vi "Test.vi"   [LabVIEW 2018]
doc: "This VI is called when test mode begins, and will automatically be terminated when it ends. You can add manual or automatic tests and invoke them from the dashboard."
uses:
  <vilib>/Rock Robotics/WPI/ThirdParty/Sensors/navX/_TypeDefs/FRIC_navX_DeviceNumbersTypeDef.ctl
  <vilib>/Rock Robotics/WPI/Utilities/WPI_GetSetVariantRefNum.vi
  <vilib>/Rock Robotics/Network Tables/NT Write Boolean.vi
  Robot Global Data.vi
  <vilib>/Rock Robotics/WPI/RobotDrive/WPI_RobotDriveMecanumDrive_Cartesian.vi
  <vilib>/Rock Robotics/WPI/ThirdParty/Phoenix-LabVIEW/Motor Controller/Get/CTRE_Phoenix_MotorController_GetQuadratureData.vi
  <vilib>/Rock Robotics/WPI/ThirdParty/Sensors/navX/_Processing Loop/FRIC_navX_Internal_Serial_ProcessingLoop.vi
types:
  T1 = typedef "FRIC_navX_DeviceNumbersTypeDef.ctl" = enum16{"Dev0", "Dev1", "Dev2", "Dev3"}
  T2 = cluster{"Yaw":dbl, "Roll":dbl, "Pitch":dbl, "Heading":dbl, "Fused Heading":dbl}
  T3 = typedef "WPI_JoystickDevRef.ctl" = cluster{"Device":T4}
  T4 = typedef "WPI_JoystickDeviceEnum.ctl" = enum16{"USB 0", "USB 1", "USB 2", "USB 3", "USB 4", "USB 5"}
  T5 = typedef "WPI_RobotDriveDevRef.ctl" = cluster{"DevStatus":errorcluster, "Motors[]":T6[], "Square Inputs":bool, "Max Output":dbl}
  T6 = typedef "WPI_MotorControlDeviceRef.ctl" = cluster{"DeviceStatus":errorcluster, "Type":T7, "PWM":cluster{"PWM Channel":T8, "DeadBand":T9}, "CAN":cluster{"Device Number":u8, "SetOutput VI Ref":variant, "GetOutput VI Ref":variant, "Enable VI Ref":variant, "Disable VI Ref":variant, "Data":variant}, "Invert":bool, "DIO PWM":cluster{"PWM \"Enable\" Channel":T8, "DIOChannel":T10, "PWM Rate":dbl}}
  T7 = typedef "WPI_MotorControlType.ctl" = enum16{"PWM", "CAN", "DIO PWM"}
  T8 = typedef "FPGA_DIOPWMChannel.ctl" = enum8{"PWM 0", "PWM 1", "PWM 2", "PWM 3", "PWM 4", "PWM 5", "PWM 6", "PWM 7", "PWM 8", "PWM 9", "PWM MXP 0", "PWM MXP 1", "PWM MXP 2", "PWM MXP 3", "PWM MXP 4", "PWM MXP 5", "PWM MXP 6", "PWM MXP 7", "PWM MXP 8", "PWM MXP 9", "Invalid"}
  T9 = typedef "WPI_PWMDeadband.ctl" = cluster{"Name":string, "maxPositivePwm":i32, "minPositivePwm":i32, "centerPwm":i32, "maxNegativePwm":i32, "minNegativePwm":i32, "angularRange":u16}
  T10 = typedef "FPGA_DIOChannel.ctl" = enum8{"DIO 0", "DIO 1", "DIO 2", "DIO 3", "DIO 4", "DIO 5", "DIO 6", "DIO 7", "DIO 8", "DIO 9", "DIO MXP 0", "DIO MXP 1", "DIO MXP 2", "DIO MXP 3", "DIO MXP 4", "DIO MXP 5", "DIO MXP 6", "DIO MXP 7", "DIO MXP 8", "DIO MXP 9", "DIO MXP 10", "DIO MXP 11", "DIO MXP 12", "DIO MXP 13", "DIO MXP 14", "DIO MXP 15", "SPI Port CS1", "SPI Port CS2", "SPI Port CS3", "SPI Port MISO", "SPI Port MOSI", "Invalid"}
  T11 = typedef "WPI_SwitchDevRef.ctl" = cluster{"DevStatus":errorcluster, "DIO Channel":T10, "CntIndex":T12, "Normally Closed":bool}
  T12 = typedef "FPGA_CounterCtrSystemIndex.ctl" = enum8{"Ctr 0", "Ctr 1", "Ctr 2", "Ctr 3", "Ctr 4", "Ctr 5", "Ctr 6", "Ctr 7", "Invalid"}
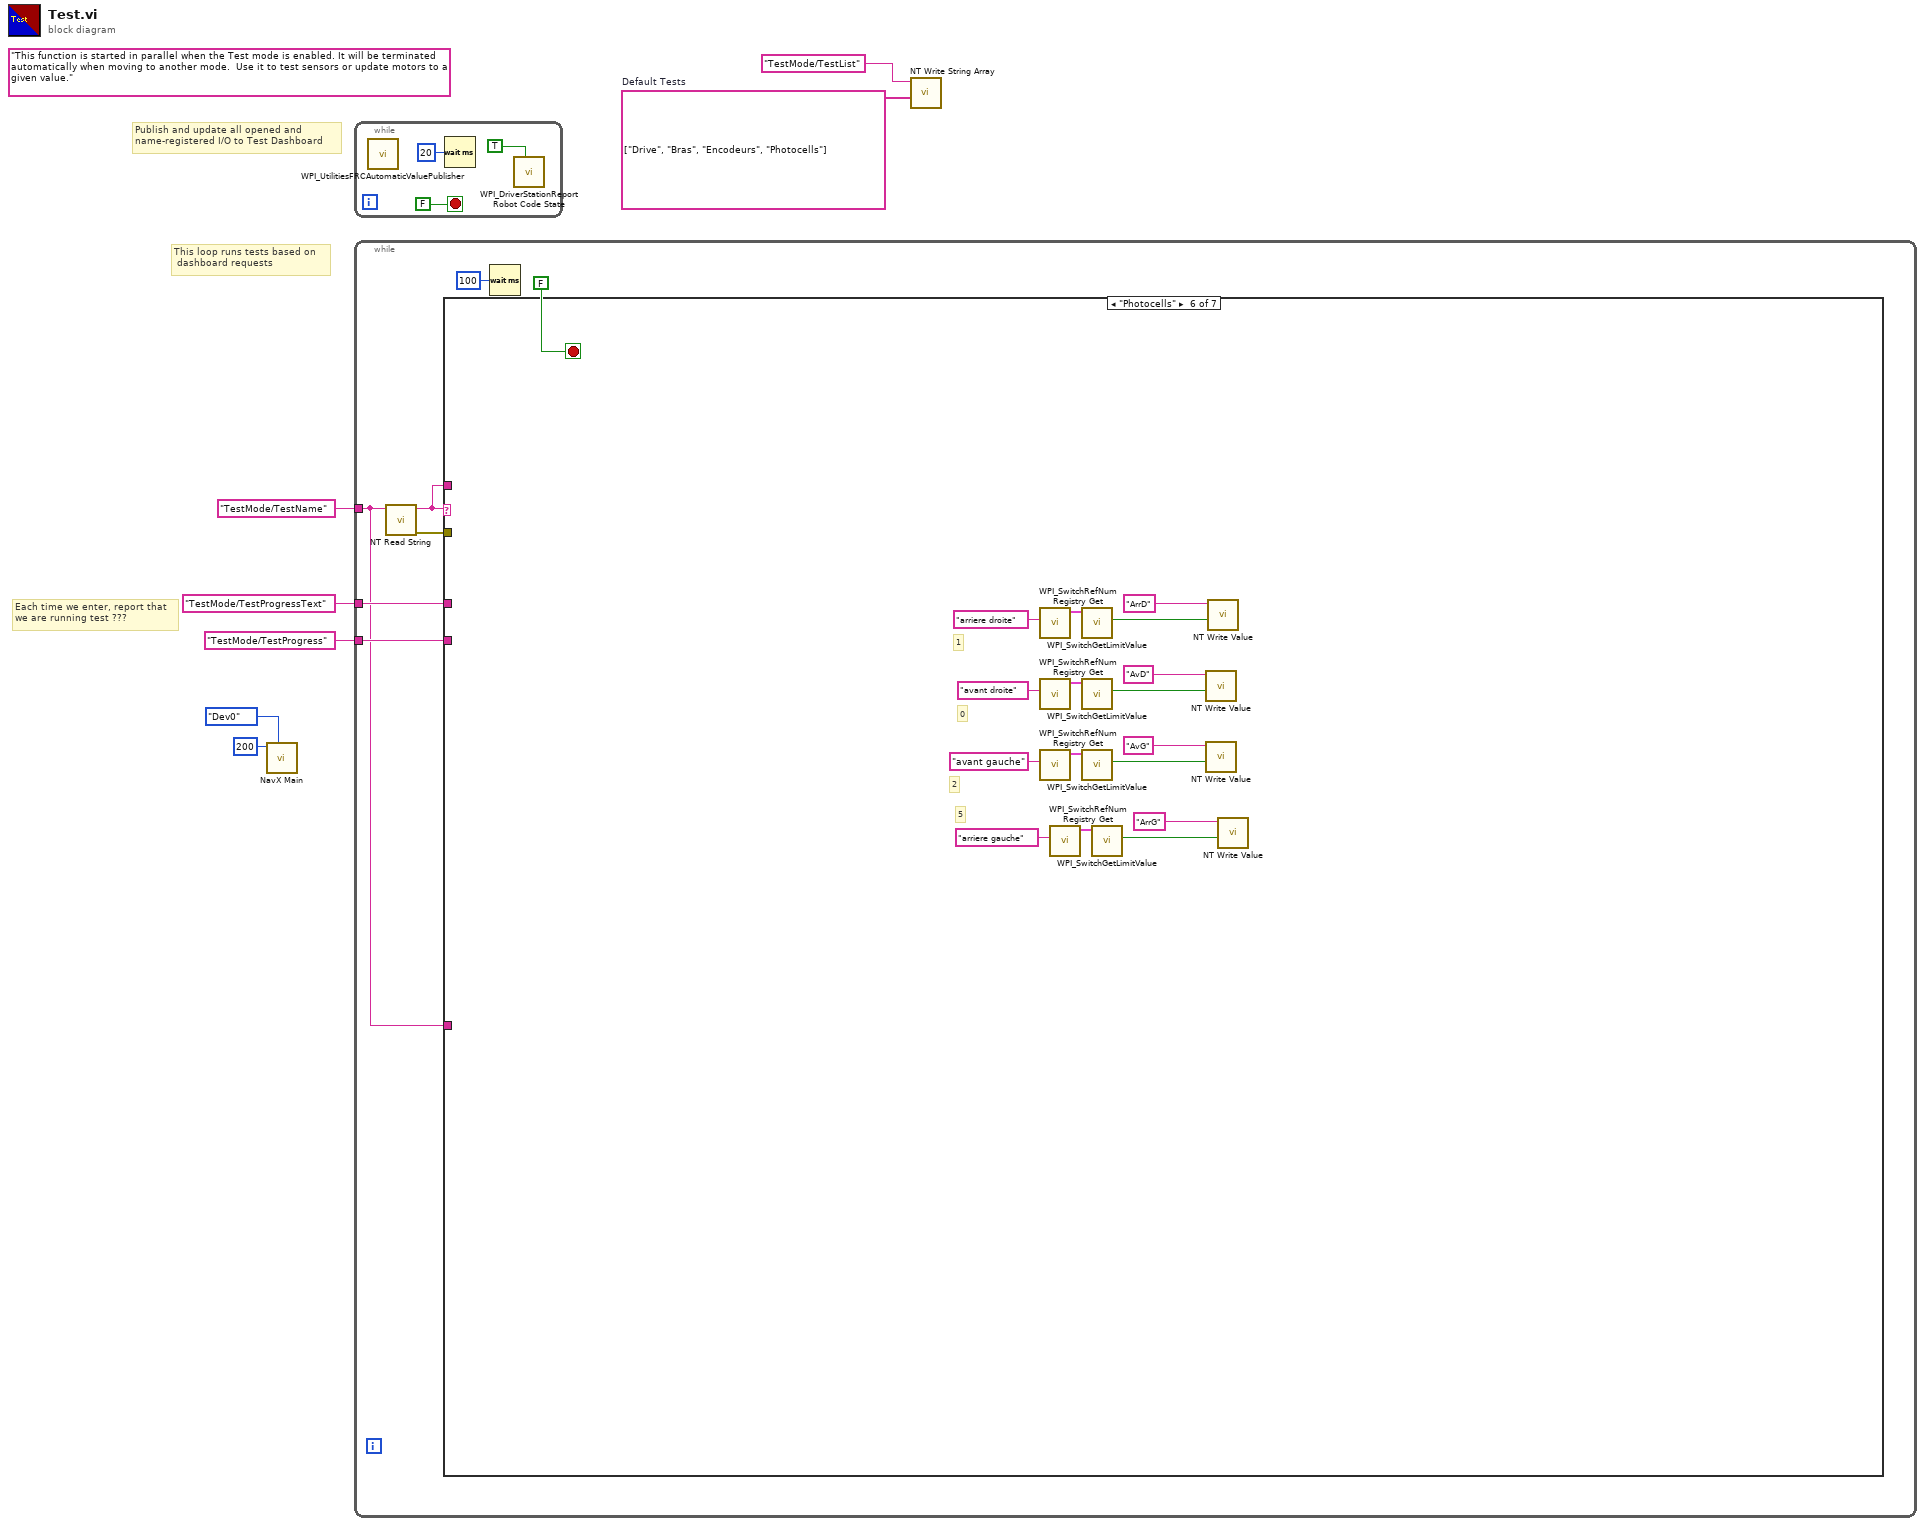
[diagram p0: block diagram]
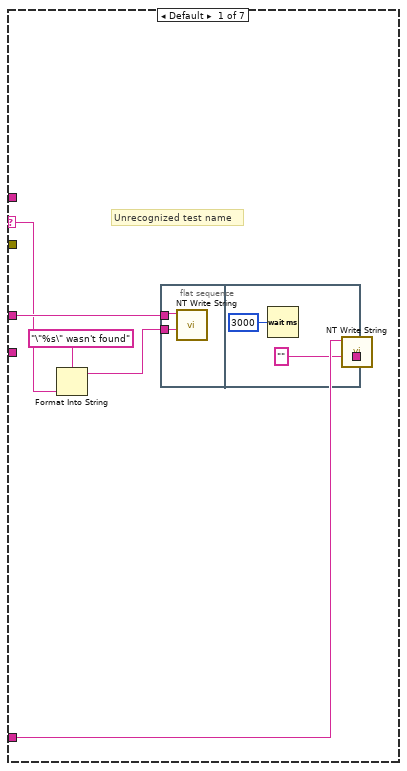
[diagram p2: hidden frame]
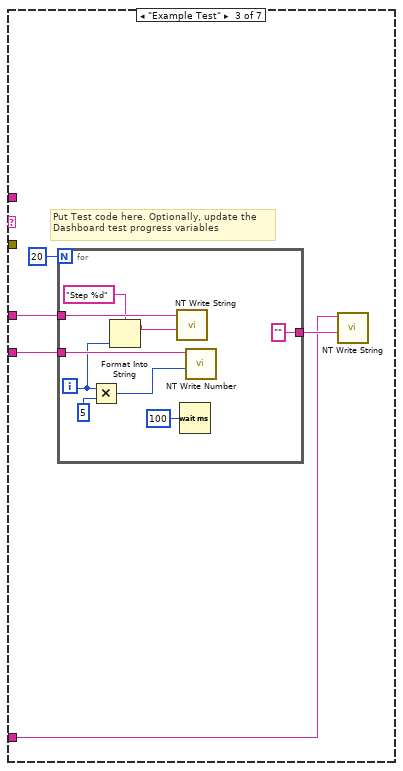
[diagram p4: hidden frame]
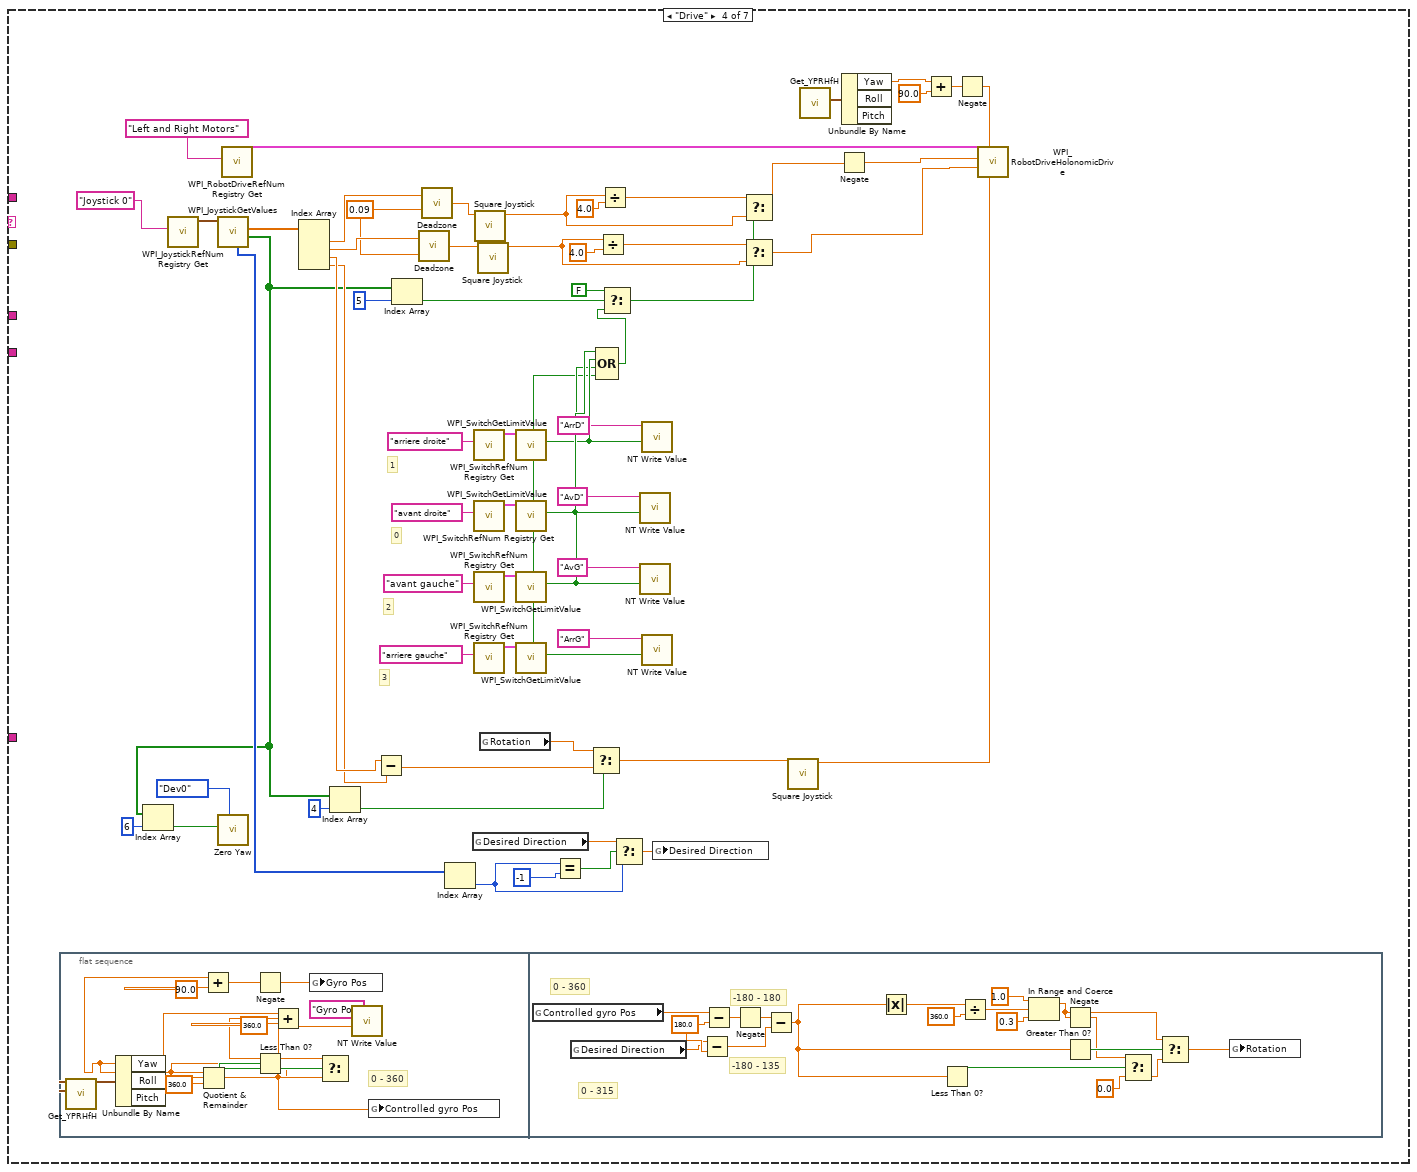
[diagram p5: hidden frame]
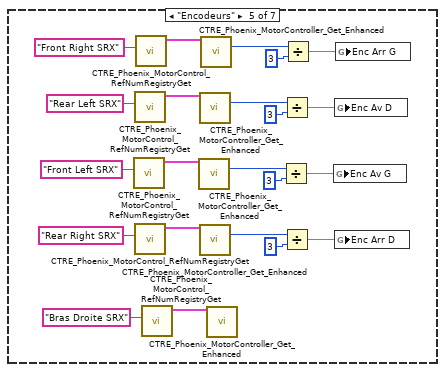
[diagram p6: hidden frame]
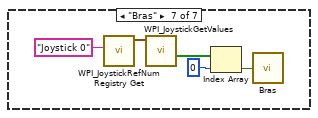
[diagram p7: hidden frame]
diagram:
  w4 = string[] ["Drive", "Bras", "Encodeurs", "Photocells"]  # Default Tests
  (unwired) "This function is started in parallel when the Test mode is enabled. It will be terminated automatically when moving to another mode.  Use it to test sensors or update motors to a given value."
  # "This loop runs tests based on \n dashboard requests"
  # "Publish and update all opened and\nname-registered I/O to Test Dashboard"
  # "Each time we enter, report that\nwe are running test ???"
  n1 = call-poly <vilib>:"NavX Main.vi"("Device Number"=FRIC_navX_DeviceNumbersTypeDef."Dev0", "Rate (4Hz-200Hz)"=u8 200) -> ()  [unwired: 10 in]
  n2 = while {
    stop <- FALSE stop-if-true
    n3 = call <vilib>:"WPI_UtilitiesFRCAutomaticValuePublisher.vi"() -> ()  [unwired: 12 in]
    n4 = Wait (ms)(milliseconds to wait=u32 20) -> ()  [unwired: 1 out]
    n5 = call <vilib>:"WPI_DriverStationReport Robot Code State.vi"("Test"=TRUE ("Autonomous")) -> ()  [unwired: 10 in, 1 out]
  }
  n6 = while {
    tunnel: "TestMode/TestName" ("Name") -> [w12]
    tunnel: "TestMode/TestProgressText" ("Name") -> [w15]
    tunnel: "TestMode/TestProgress" ("Name") -> [w14]
    stop <- FALSE stop-if-true
    n7 = call <vilib>:"NT Read String.vi"("Name"=w12) -> ("error out"=w11:errorcluster, "String"=w13:string)  [unwired: 9 in]
    n8 = case shown="\"Photocells\"" w13 {
      selector: w13 -> [w22 _ _ _ _ _ _]
      tunnel: w12 -> [w19 _ w28 _ _ _ _]
      tunnel: w15 -> [w23 _ w31 _ _ _ _]
      tunnel: w14 -> [_ _ w32 _ _ _ _]
      tunnel: w13 -> [_ _ _ _ _ _ _]
      tunnel: w11 -> [_ _ _ _ _ _ _]
      frame Default {
        # "Unrecognized test name"
        n9 = Format Into String(format string="\"%s\" wasn't found" ("Name"), w22) -> (resulting string=w21:string)  [unwired: 2 in, 1 out]
        n10 = flat-sequence {
          tunnel: w23 -> [w24]
          tunnel: w21 -> [w25]
          tunnel: ["" ("Name")] -> w18
          frame #0 {
            n11 = call <vilib>:"NT Write String.vi"("String"=w25, "Name"=w24) -> ()  [unwired: 9 in, 1 out]
          }
          frame #1 {
            n12 = Wait (ms)(milliseconds to wait=u32 3000) -> ()  [unwired: 1 out]
          }
        }
        n13 = call <vilib>:"NT Write String.vi"("String"=w18, "Name"=w19) -> ()  [unwired: 9 in, 1 out]
      }
      frame "" {
        # "No test to run"
      }
      frame "Example Test" {
        # "Put Test code here. Optionally, update the\nDashboard test progress variables"
        n14 = for {
          N: 20 -> [_]
          tunnel: w32 -> [w41]
          tunnel: w31 -> [w39]
          tunnel: ["" ("String")] -> w29
          i -> [w36]
          n15 = Multiply(x=w36, y=u32 5 ("milliseconds to wait")) -> (x*y=w37:u32)
          n16 = Format Into String(format string="Step %d", w36) -> (resulting string=w34:string)  [unwired: 2 in, 1 out]
          n17 = call <vilib>:"NT Write String.vi"("String"=w34, "Name"=w39) -> ()  [unwired: 9 in, 1 out]
          n18 = Wait (ms)(milliseconds to wait=u32 100) -> ()  [unwired: 1 out]
          n19 = call <vilib>:"NT Write Number.vi"("Numeric"=w37, "Name"=w41) -> ()  [unwired: 9 in, 1 out]
        }
        n20 = call <vilib>:"NT Write String.vi"("String"=w29, "Name"=w28) -> ()  [unwired: 9 in, 1 out]
      }
      frame "Drive" {
        w86 = 0.09 ("DeadZone")
        # "3"
        # "2"
        # "1"
        # "0"
        n21 = flat-sequence {
          frame #0 {
            # "0 - 360"
            n22 = call <vilib>:"Get_YPRHfH.vi"() -> ("YRPHfH"=w116:T2)  [unwired: 11 in]
            n23 = Unbundle By Name(w116) -> ("Yaw"=w105:dbl)  [unwired: 2 out]
            n24 = Quotient & Remainder(x=w105, y=360.0) -> (x-y*floor(x/y)=w111:dbl)  [unwired: 1 out]
            n25 = Add(x=w105, y=90.0) -> (x+y=w106:dbl)
            n26 = Negate(x=w106) -> (-x=w108:dbl)
            n27 = Less Than 0?(x=w111) -> (x < 0?=w112:bool)
            n28 = Add(x=w111, y=360.0) -> (x+y=w110:dbl)
            n29 = global write "Robot Global Data.vi" "Gyro Pos"(w108) -> ()
            n30 = Select(t=w110, s=w112, f=w111) -> (s? t:f=w109:dbl)
            n31 = call-poly <vilib>:"NT Write Value.vi"("Numeric"=w109, "Name"="Gyro Pos") -> ()  [unwired: 9 in, 1 out]
            n32 = global write "Robot Global Data.vi" "Controlled gyro Pos"(w109) -> ()
          }
          frame #1 {
            w118 = 180.0 ("y")
            # "-180 - 135"
            # "-180 - 180"
            # "0 - 315"
            # "0 - 360"
            n33 = global read "Robot Global Data.vi" "Controlled gyro Pos"() -> (w122:dbl)
            n34 = global read "Robot Global Data.vi" "Desired Direction"() -> (w117:dbl)
            n35 = Subtract(x=w117, y=w118) -> (x-y=w119:dbl)
            n36 = Subtract(x=w122, y=w118) -> (x-y=w121:dbl)
            n37 = Negate(x=w121) -> (-x=w120:dbl)
            n38 = Subtract(x=w120, y=w119) -> (x-y=w124:dbl)
            n39 = Absolute Value(x=w124) -> (abs(x)=w135:dbl)
            n40 = Less Than 0?(x=w124) -> (x < 0?=w126:bool)
            n41 = Divide(x=w135, y=360.0) -> (x/y=w133:dbl)
            n42 = In Range and Coerce(upper limit=1.0, x=w133, lower limit=0.3) -> (coerced(x)=w128:dbl)  [unwired: 1 out]
            n43 = Negate(x=w128) -> (-x=w127:dbl)
            n44 = Greater Than 0?(x=w124) -> (x > 0?=w129:bool)
            n45 = Select(t=w127, s=w126, f=0.0) -> (s? t:f=w130:dbl)
            n46 = Select(t=w128, s=w129, f=w130) -> (s? t:f=w123:dbl)
            n47 = global write "Robot Global Data.vi" "Rotation"(w123) -> ()
          }
        }
        n48 = call <vilib>:"WPI_JoystickRefNum Registry Get.vi"("refnum name"="Joystick 0") -> ("JoystickDevRef"=w102:T3)  [unwired: 1 in, 9 out]
        n49 = call <vilib>:"WPI_JoystickGetValues.vi"("JoystickDevRef"=w102) -> ("Buttons"=w59:bool[], "Axes"=w101:dbl[], "POVs"=w60:i16[])  [unwired: 6 in, 2 out]
        n50 = Index Array(array=w59, index=6) -> (element=w62:bool)
        n51 = call <vilib>:"Zero Yaw.vi"("Device Number"=FRIC_navX_DeviceNumbersTypeDef."Dev0", "Zero"=w62) -> ()  [unwired: 10 in]
        n52 = call <vilib>:"WPI_RobotDriveRefNum Registry Get.vi"("refnum name"="Left and Right Motors") -> ("RobotDriveDevRef"=w100:T5)  [unwired: 1 in, 9 out]
        n53 = Index Array(array=w101) -> (element #1=w99:dbl, element #2=w98:dbl, element #3=w77:dbl, element #4=w76:dbl)  [unwired: 4 in]
        n54 = Index Array(array=w59, index=4) -> (element=w96:bool)
        n55 = Subtract(x=w77, y=w76) -> (x-y=w94:dbl)
        n56 = Index Array(array=w59, index=5) -> (element=w92:bool)
        n57 = call "Deadzone.vi"("DeadZone"=w86, "In"=w98) -> ("Out"=w81:dbl)
        n58 = call "Deadzone.vi"("DeadZone"=w86, "In"=w99) -> ("Out"=w79:dbl)
        n59 = Index Array(array=w60) -> (element=w64:i16)  [unwired: 1 in]
        n60 = global read "Robot Global Data.vi" "Desired Direction"() -> (w66:dbl)
        n61 = call <vilib>:"WPI_SwitchRefNum Registry Get.vi"("refnum name"="arriere droite") -> ("SwitchDevRef"=w54:T11)  [unwired: 9 in, 1 out]
        n62 = call <vilib>:"WPI_SwitchRefNum Registry Get.vi"("refnum name"="avant droite") -> ("SwitchDevRef"=w55:T11)  [unwired: 9 in, 1 out]
        n63 = call <vilib>:"WPI_SwitchRefNum Registry Get.vi"("refnum name"="avant gauche") -> ("SwitchDevRef"=w53:T11)  [unwired: 9 in, 1 out]
        n64 = call <vilib>:"WPI_SwitchRefNum Registry Get.vi"("refnum name"="arriere gauche") -> ("SwitchDevRef"=w45:T11)  [unwired: 9 in, 1 out]
        n65 = call "Square Joystick.vi"("In"=w79) -> ("Squared Output"=w78:dbl)  [unwired: 10 in]
        n66 = call "Square Joystick.vi"("In"=w81) -> ("Squared Output"=w80:dbl)  [unwired: 10 in]
        n67 = global read "Robot Global Data.vi" "Rotation"() -> (w95:dbl)
        n68 = call <vilib>:"WPI_SwitchGetLimitValue.vi"("SwitchDevRef"=w54) -> ("Switch Pressed"=w51:bool)  [unwired: 8 in, 2 out]
        n69 = call <vilib>:"WPI_SwitchGetLimitValue.vi"("SwitchDevRef"=w55) -> ("Switch Pressed"=w52:bool)  [unwired: 8 in, 2 out]
        n70 = call <vilib>:"WPI_SwitchGetLimitValue.vi"("SwitchDevRef"=w53) -> ("Switch Pressed"=w50:bool)  [unwired: 8 in, 2 out]
        n71 = call <vilib>:"WPI_SwitchGetLimitValue.vi"("SwitchDevRef"=w45) -> ("Switch Pressed"=w43:bool)  [unwired: 8 in, 2 out]
        n72 = Equal?(x=w64, y=i16 -1) -> (x = y?=w67:bool)
        n73 = Select(t=w95, s=w96, f=w94) -> (s? t:f=w75:dbl)
        n74 = Compound Arithmetic op=OR(w52, w51, w50, w43) -> (w42:bool)
        n75 = Divide(x=w80, y=4.0) -> (x/y=w87:dbl)
        n76 = Divide(x=w78, y=4.0) -> (x/y=w89:dbl)
        n77 = Select(t=FALSE, s=w92, f=w42) -> (s? t:f=w84:bool)
        n78 = Select(t=w66, s=w67, f=w64) -> (s? t:f=w65:dbl)
        n79 = call-poly <vilib>:"NT Write Value.vi"("Boolean"=w52, "Name"="AvD") -> ()  [unwired: 9 in, 1 out]
        n80 = call-poly <vilib>:"NT Write Value.vi"("Boolean"=w50, "Name"="AvG") -> ()  [unwired: 9 in, 1 out]
        n81 = call-poly <vilib>:"NT Write Value.vi"("Boolean"=w51, "Name"="ArrD") -> ()  [unwired: 9 in, 1 out]
        n82 = call-poly <vilib>:"NT Write Value.vi"("Boolean"=w43, "Name"="ArrG") -> ()  [unwired: 9 in, 1 out]
        n83 = global write "Robot Global Data.vi" "Desired Direction"(w65) -> ()
        n84 = Select(t=w89, s=w84, f=w78) -> (s? t:f=w83:dbl)
        n85 = Select(t=w87, s=w84, f=w80) -> (s? t:f=w82:dbl)
        n86 = call "Square Joystick.vi"("In"=w75) -> ("Squared Output"=w74:dbl)  [unwired: 10 in]
        n87 = call <vilib>:"Get_YPRHfH.vi"() -> ("YRPHfH"=w73:T2)  [unwired: 11 in]
        n88 = Negate(x=w83) -> (-x=w85:dbl)
        n89 = Unbundle By Name(w73) -> ("Yaw"=w69:dbl)  [unwired: 2 out]
        n90 = Add(x=w69, y=90.0) -> (x+y=w71:dbl)
        n91 = Negate(x=w71) -> (-x=w70:dbl)
        n92 = call-poly <vilib>:"WPI_RobotDriveHolonomicDrive.vi"("Rotation"=w74, "Gyro Angle"=w70, "Y"=w82, "X"=w85, "RobotDriveDevRef"=w100) -> ()  [unwired: 4 in, 3 out]
      }
      frame "Encodeurs" {
        n93 = call <vilib>:"CTRE_Phoenix_MotorControl_RefNumRegistryGet.vi"("refnum name"="Front Left SRX") -> ("PhoenixMotorControlDevRef"=w139:T6)  [unwired: 9 in, 1 out]
        n94 = call <vilib>:"CTRE_Phoenix_MotorControl_RefNumRegistryGet.vi"("refnum name"="Rear Left SRX") -> ("PhoenixMotorControlDevRef"=w140:T6)  [unwired: 9 in, 1 out]
        n95 = call <vilib>:"CTRE_Phoenix_MotorControl_RefNumRegistryGet.vi"("refnum name"="Rear Right SRX") -> ("PhoenixMotorControlDevRef"=w138:T6)  [unwired: 9 in, 1 out]
        n96 = call <vilib>:"CTRE_Phoenix_MotorControl_RefNumRegistryGet.vi"("refnum name"="Front Right SRX") -> ("PhoenixMotorControlDevRef"=w141:T6)  [unwired: 9 in, 1 out]
        n97 = call <vilib>:"CTRE_Phoenix_MotorControl_RefNumRegistryGet.vi"("refnum name"="Bras Droite SRX") -> ("PhoenixMotorControlDevRef"=w137:T6)  [unwired: 9 in, 1 out]
        n98 = call-poly <vilib>:"CTRE_Phoenix_MotorController_Get_Enhanced.vi"("PhoenixMotorControlDevRef"=w139) -> ("Quadrature Position"=w150:i32)  [unwired: 11 in, 3 out]
        n99 = call-poly <vilib>:"CTRE_Phoenix_MotorController_Get_Enhanced.vi"("PhoenixMotorControlDevRef"=w140) -> ("Quadrature Position"=w153:i32)  [unwired: 11 in, 3 out]
        n100 = call-poly <vilib>:"CTRE_Phoenix_MotorController_Get_Enhanced.vi"("PhoenixMotorControlDevRef"=w138) -> ("Quadrature Position"=w151:i32)  [unwired: 11 in, 3 out]
        n101 = call-poly <vilib>:"CTRE_Phoenix_MotorController_Get_Enhanced.vi"("PhoenixMotorControlDevRef"=w141) -> ("Quadrature Position"=w152:i32)  [unwired: 11 in, 3 out]
        n102 = call-poly <vilib>:"CTRE_Phoenix_MotorController_Get_Enhanced.vi"("PhoenixMotorControlDevRef"=w137) -> ()  [unwired: 11 in, 4 out]
        n103 = Divide(x=w150, y=3) -> (x/y=w144:dbl)
        n104 = Divide(x=w153, y=3) -> (x/y=w143:dbl)
        n105 = Divide(x=w151, y=3) -> (x/y=w145:dbl)
        n106 = Divide(x=w152, y=3) -> (x/y=w142:dbl)
        n107 = global write "Robot Global Data.vi" "Enc Av G"(w144) -> ()
        n108 = global write "Robot Global Data.vi" "Enc Av D"(w143) -> ()
        n109 = global write "Robot Global Data.vi" "Enc Arr D"(w145) -> ()
        n110 = global write "Robot Global Data.vi" "Enc Arr G"(w142) -> ()
      }
      frame "Photocells" {
        # "5"
        # "2"
        # "1"
        # "0"
        n111 = call <vilib>:"WPI_SwitchRefNum Registry Get.vi"("refnum name"="arriere droite") -> ("SwitchDevRef"=w169:T11)  [unwired: 9 in, 1 out]
        n112 = call <vilib>:"WPI_SwitchRefNum Registry Get.vi"("refnum name"="avant droite") -> ("SwitchDevRef"=w170:T11)  [unwired: 9 in, 1 out]
        n113 = call <vilib>:"WPI_SwitchRefNum Registry Get.vi"("refnum name"="avant gauche") -> ("SwitchDevRef"=w168:T11)  [unwired: 9 in, 1 out]
        n114 = call <vilib>:"WPI_SwitchRefNum Registry Get.vi"("refnum name"="arriere gauche") -> ("SwitchDevRef"=w160:T11)  [unwired: 9 in, 1 out]
        n115 = call <vilib>:"WPI_SwitchGetLimitValue.vi"("SwitchDevRef"=w169) -> ("Switch Pressed"=w166:bool)  [unwired: 8 in, 2 out]
        n116 = call <vilib>:"WPI_SwitchGetLimitValue.vi"("SwitchDevRef"=w170) -> ("Switch Pressed"=w167:bool)  [unwired: 8 in, 2 out]
        n117 = call <vilib>:"WPI_SwitchGetLimitValue.vi"("SwitchDevRef"=w168) -> ("Switch Pressed"=w165:bool)  [unwired: 8 in, 2 out]
        n118 = call <vilib>:"WPI_SwitchGetLimitValue.vi"("SwitchDevRef"=w160) -> ("Switch Pressed"=w159:bool)  [unwired: 8 in, 2 out]
        n119 = call-poly <vilib>:"NT Write Value.vi"("Boolean"=w167, "Name"="AvD") -> ()  [unwired: 9 in, 1 out]
        n120 = call-poly <vilib>:"NT Write Value.vi"("Boolean"=w165, "Name"="AvG") -> ()  [unwired: 9 in, 1 out]
        n121 = call-poly <vilib>:"NT Write Value.vi"("Boolean"=w166, "Name"="ArrD") -> ()  [unwired: 9 in, 1 out]
        n122 = call-poly <vilib>:"NT Write Value.vi"("Boolean"=w159, "Name"="ArrG") -> ()  [unwired: 9 in, 1 out]
      }
      frame "Bras" {
        n123 = call <vilib>:"WPI_JoystickRefNum Registry Get.vi"("refnum name"="Joystick 0") -> ("JoystickDevRef"=w174:T3)  [unwired: 1 in, 9 out]
        n124 = call <vilib>:"WPI_JoystickGetValues.vi"("JoystickDevRef"=w174) -> ("Buttons"=w175:bool[])  [unwired: 6 in, 4 out]
        n125 = Index Array(array=w175, index=0) -> (element=w177:bool)
        n126 = call "Bras.vi"("Commande"=w177) -> ()
      }
    }
    n127 = Wait (ms)(milliseconds to wait=u32 100) -> ()  [unwired: 1 out]
  }
  n128 = call <vilib>:"NT Write String Array.vi"("String Array"=w4, "Name"="TestMode/TestList") -> ()  [unwired: 9 in, 1 out]
